vi "Do Comparison.vi"(8 "error in (no error)":errorcluster, 10 "Compare String":string, 11 "String Filters in":refnum<class "String Filters.lvclass">) -> (0 "error out":errorcluster, 2 "Filtered":bool)   [LabVIEW 2016, in "Assert API Components.lvlib" / "String Filters.lvclass"]
uses:
  String Filters.lvclass
  String Filters.lvclass/String Filters.ctl
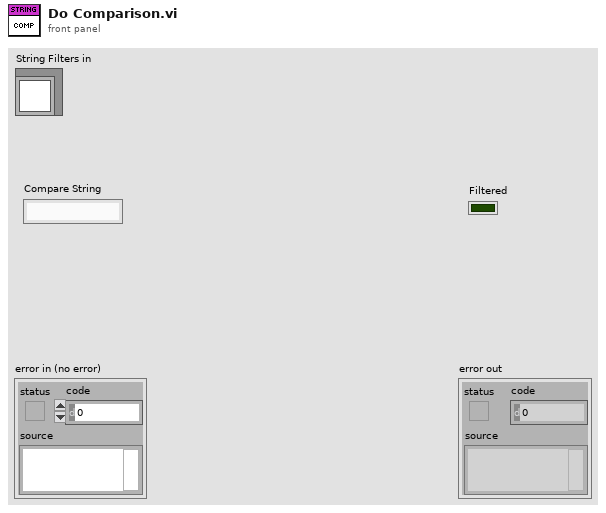
[diagram p1: front panel]
types:
  T1 = enum16{"Contains", "Does Not Contain", "Starts With", "Equals", "Does Not Equal"}
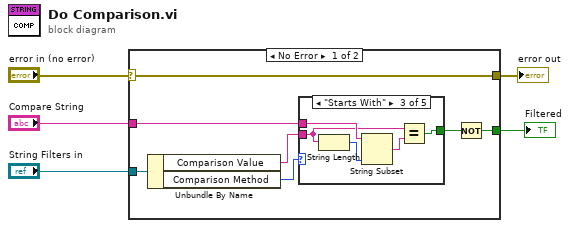
[diagram p0: block diagram]
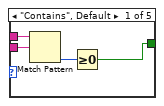
[diagram p2: hidden frame]
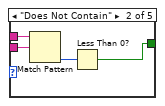
[diagram p3: hidden frame]
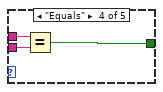
[diagram p4: hidden frame]
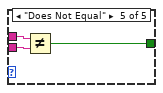
[diagram p5: hidden frame]
diagram:
  n1 = case shown="No Error" "error in (no error)" {
    selector: "error in (no error)" -> [w12 w32]
    tunnel: [w12 w32] -> w4
    tunnel: "String Filters in" -> [w11 _]
    tunnel: "Compare String" -> [w10 _]
    tunnel: [w7 _] -> w1
    frame No Error {
      n2 = Unbundle By Name(w11) -> ("Comparison Value"=w9:string, "Comparison Method"=w6:T1)
      n3 = case shown="\"Starts With\"" w6 {
        tunnel: w10 -> [w16 w20 w25 w27 w30]
        tunnel: w9 -> [w15 w19 w22 w28 w31]
        tunnel: [w13 w17 w21 w26 w29] -> w8
        frame "Contains", Default {
          n4 = Match Pattern(string=w16, regular expression=w15) -> (offset past match=w14:i32)  [unwired: 1 in, 3 out]
          n5 = Greater Or Equal To 0?(x=w14) -> (x >= 0?=w13:bool)
        }
        frame "Does Not Contain" {
          n6 = Match Pattern(string=w20, regular expression=w19) -> (offset past match=w18:i32)  [unwired: 1 in, 3 out]
          n7 = Less Than 0?(x=w18) -> (x < 0?=w17:bool)
        }
        frame "Starts With" {
          n8 = String Length(string=w22) -> (length=w24:i32)
          n9 = String Subset(string=w25, length (rest)=w24) -> (substring=w23:string)  [unwired: 1 in]
          n10 = Equal?(x=w22, y=w23) -> (x = y?=w21:bool)
        }
        frame "Equals" {
          n11 = Equal?(x=w27, y=w28) -> (x = y?=w26:bool)
        }
        frame "Does Not Equal" {
          n12 = Not Equal?(x=w30, y=w31) -> (x != y?=w29:bool)
        }
      }
      n13 = Not(x=w8) -> (.not. x?=w7:bool)
    }
    frame Error {
    }
  }
  "error out" <- w4
  "Filtered" <- w1
